vi "PPL CD XML Updater.vi"(5 "Files Generated by Build":path[](array[path]), 6 "Top Level/Always Included VIs":path[](array[path]), 7 "Destination Path":path, 8 "error in (no error)":errorcluster, 9 "Target Name":string, 10 "Build Specification Name":string, 11 "Project Path":path) -> (0 "error out":errorcluster)   [LabVIEW 2019]
doc: "This VI is called after each run of a build specification. The VI will copy the generated LLB (Engine or System Explorer) into the VeriStand Custom Device folder (...\\Documents\\National Instruments\\NI VeriStand 2013...)."
uses:
  LVLIBP CD XML Updater/LVLIBP CD XML Updater.lvlib
  LVLIBP CD XML Updater/Project XML Editor/Project XML Editor.lvclass
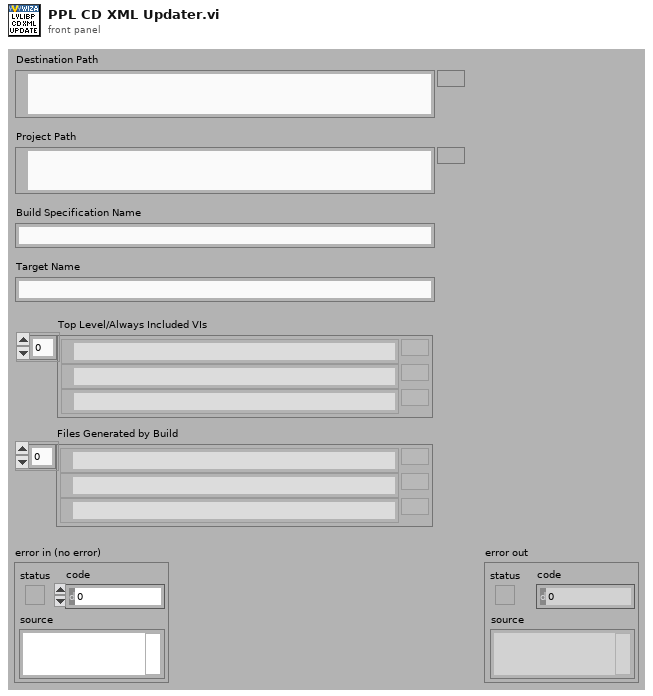
[diagram p1: front panel]
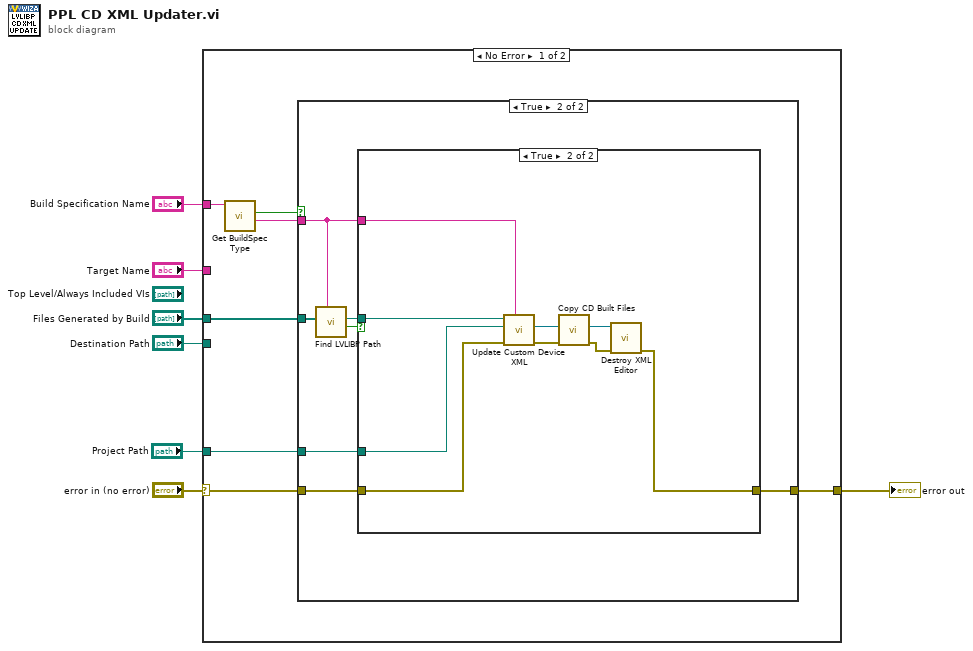
[diagram p0: block diagram]
diagram:
  n1 = case shown="No Error" "error in (no error)" {
    selector: "error in (no error)" -> [w11 w33]
    tunnel: [w8 w33] -> w5
    tunnel: "Project Path" -> [w10 _]
    tunnel: "Files Generated by Build" -> [w9 _]
    tunnel: "Target Name" -> [_ _]
    tunnel: "Build Specification Name" -> [w14 _]
    tunnel: "Destination Path" -> [_ _]
    frame No Error {
      n2 = call "Get BuildSpec Type.vi"("Build Specification Name in"=w14) -> ("Build Spec Type"=w12:string, "Found ?"=w13:bool)  [unwired: 8 in, 1 out]
      n3 = case shown="True" w13 {
        tunnel: w12 -> [_ w20]
        tunnel: w11 -> [w15 w17]
        tunnel: w10 -> [_ w18]
        tunnel: [w15 w16] -> w8
        tunnel: w9 -> [_ w19]
        frame False {
        }
        frame True {
          n4 = call "Find LVLIBP Path.vi"("Build Type"=w20, "Files Generated by Build"=w19) -> ("Found ?"=w21:bool, "Packed Library Path"=w22:path)  [unwired: 8 in]
          n5 = case shown="True" w21 {
            tunnel: w22 -> [_ w31]
            tunnel: w20 -> [_ w29]
            tunnel: w18 -> [_ w32]
            tunnel: w17 -> [w23 w30]
            tunnel: [w23 w26] -> w16
            frame False {
            }
            frame True {
              n6 = call "Update Custom Device XML.vi"("Build Spec Type"=w29, "error in (no error)"=w30, "CD XML/Project Path"=w32, "Packed Library Path"=w31) -> ("error out"=w28:errorcluster, "Project XML Editor out"=w25:refnum<class "Project XML Editor.lvclass">)  [unwired: 6 in]
              n7 = call "Copy CD Built Files.vi"("error in (no error)"=w28, "Project XML Editor in"=w25) -> ("error out"=w27:errorcluster, "Project XML Editor out"=w24:refnum<class "Project XML Editor.lvclass">)  [unwired: 8 in]
              n8 = call "Destroy XML Editor.vi"("error in (no error)"=w27, "Project XML Editor in"=w24) -> ("error out"=w26:errorcluster)  [unwired: 9 in]
            }
          }
        }
      }
    }
    frame Error {
    }
  }
  "error out" <- w5
